vi "DAQ signal generation vi2.vi"(6 "Time for each step":dbl, 9 "Total time":dbl, 10 "DAQ1":waveform(dbl)[](array[waveform]), 11 "DAQ 2":waveform(dbl)[](array[waveform])) -> (0 "error out":errorcluster, 3 "error out 7":errorcluster)   [LabVIEW 2016]
uses:
  <vilib>/DAQmx/write.llb/DAQmx Write (Analog 1D Wfm NChan NSamp).vi
  <vilib>/DAQmx/create/channels.llb/DAQmx Create Channel (AO-Voltage-Basic).vi
  <vilib>/DAQmx/configure/timing.llb/DAQmx Timing (Sample Clock).vi
  <vilib>/DAQmx/miscellaneous.llb/DAQmx Fill In Error Info.vi
  <vilib>/DAQmx/configure/trigger.llb/DAQmx Start Trigger (Digital Edge).vi
  <resource>/objmgr/daqmx.rc
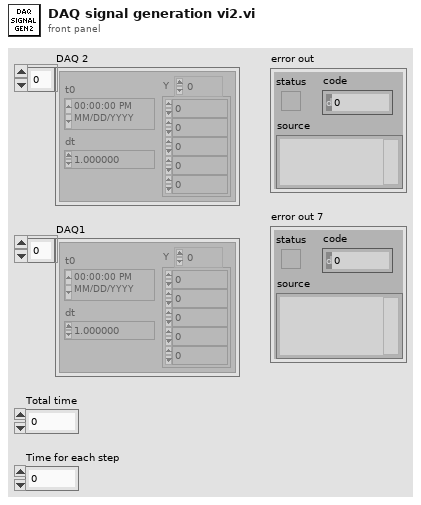
[diagram p1: front panel]
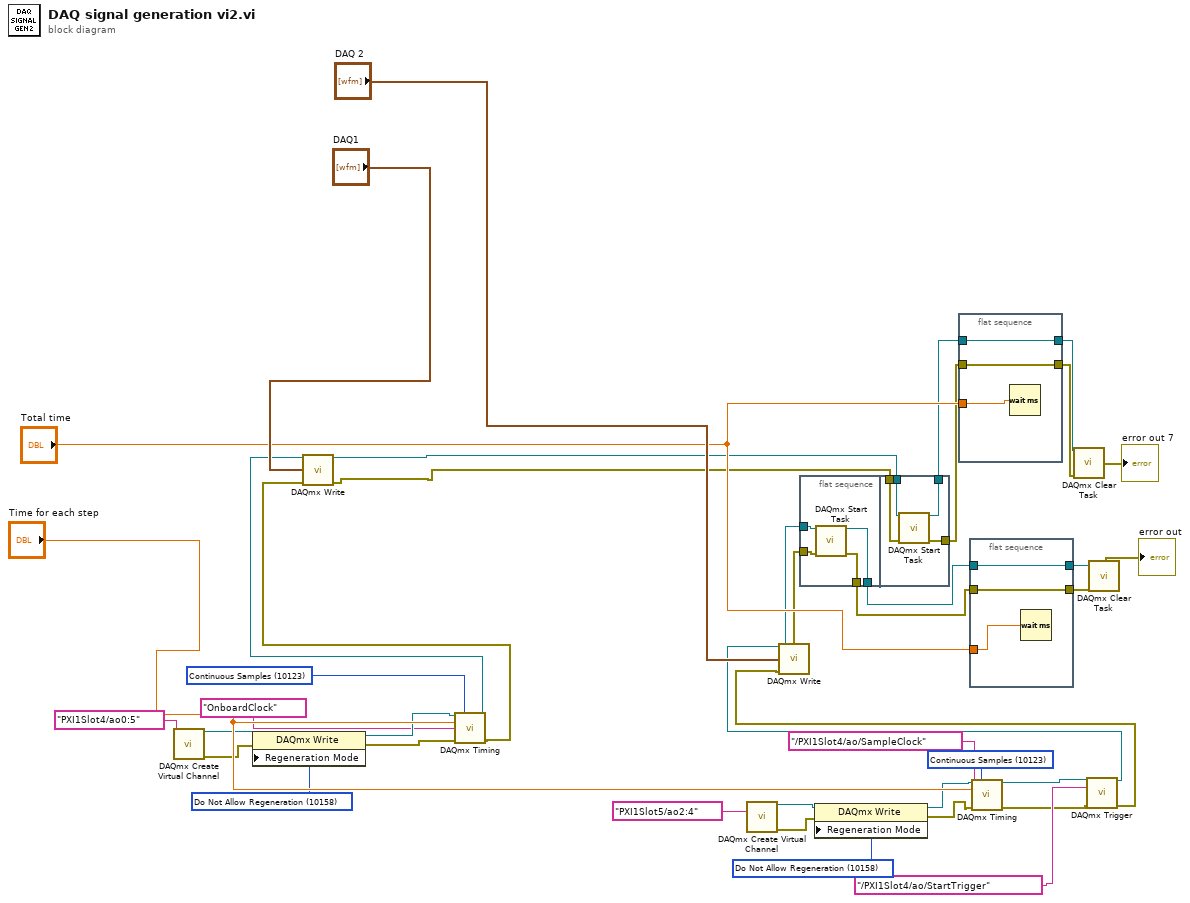
[diagram p0: block diagram]
diagram:
  w37 = 10158 items=["Allow Regeneration"=10097, "Do Not Allow Regeneration"=10158] ("RegenMode")
  w11 = 10158 items=["Allow Regeneration"=10097, "Do Not Allow Regeneration"=10158] ("RegenMode")
  w10 = 10123 items=["Finite Samples"=10178, "Continuous Samples"=10123, "Hardware Timed Single Point"=12522] ("sample mode")
  w4 = 10123 items=["Finite Samples"=10178, "Continuous Samples"=10123, "Hardware Timed Single Point"=12522] ("sample mode")
  n1 = call-poly <vilib>:"DAQmx Create Virtual Channel.vi"("physical channels"=tag "PXI1Slot4/ao0:5") -> ("task out"=w35:refnum<k21>, "error out"=w36:errorcluster)  [unwired: 13 in]
  n2 = property class="DAQmx Write"(reference=w35, error in=w36, "Regeneration Mode"=w37) -> (reference out=w33:refnum<k21>, error out=w34:errorcluster)
  n3 = call-poly <vilib>:"DAQmx Timing.vi"("task/channels in"=w33, "sample mode"=w4, "rate"="Time for each step", "source"=tag "OnboardClock", "error in"=w34) -> ("task out"=w5:refnum<k21>, "error out"=w32:errorcluster)  [unwired: 9 in]
  n4 = call-poly <vilib>:"DAQmx Write.vi"("task/channels in"=w5, "data"="DAQ1", "error in"=w32) -> ("task out"=w26:refnum<k21>, "error out"=w27:errorcluster)  [unwired: 10 in, 1 out]
  n5 = call-poly <vilib>:"DAQmx Create Virtual Channel.vi"("physical channels"=tag "PXI1Slot5/ao2:4") -> ("task out"=w6:refnum<k21>, "error out"=w7:errorcluster)  [unwired: 13 in]
  n6 = flat-sequence {
    tunnel: w17 -> [w45]
    tunnel: w18 -> [w44]
    tunnel: [w43] -> w23
    tunnel: [w42] -> w24
    tunnel: w26 -> [w49]
    tunnel: w27 -> [w48]
    tunnel: [w47] -> w28
    tunnel: [w46] -> w31
    frame #0 {
      n7 = call <vilib>:"DAQmx Start Task.vi"("task/channels in"=w44, "error in"=w45) -> ("task out"=w42:refnum<k21>, "error out"=w43:errorcluster)  [unwired: 12 in]
    }
    frame #1 {
      n8 = call <vilib>:"DAQmx Start Task.vi"("task/channels in"=w49, "error in"=w48) -> ("task out"=w47:refnum<k21>, "error out"=w46:errorcluster)  [unwired: 12 in]
    }
  }
  n9 = property class="DAQmx Write"(reference=w6, error in=w7, "Regeneration Mode"=w11) -> (reference out=w8:refnum<k21>, error out=w9:errorcluster)
  n10 = flat-sequence {
    tunnel: w31 -> [w51]
    tunnel: w28 -> [w52]
    tunnel: [w52] -> w29
    tunnel: [w51] -> w30
    tunnel: "Total time" -> [w50]
    frame #0 {
      n11 = Wait (ms)(milliseconds to wait=w50) -> ()  [unwired: 1 out]
    }
  }
  n12 = flat-sequence {
    tunnel: w23 -> [w54]
    tunnel: w24 -> [w55]
    tunnel: [w55] -> w19
    tunnel: [w54] -> w20
    tunnel: "Total time" -> [w53]
    frame #0 {
      n13 = Wait (ms)(milliseconds to wait=w53) -> ()  [unwired: 1 out]
    }
  }
  n14 = call-poly <vilib>:"DAQmx Timing.vi"("task/channels in"=w8, "sample mode"=w10, "rate"="Time for each step", "source"=tag "/PXI1Slot4/ao/SampleClock", "error in"=w9) -> ("task out"=w12:refnum<k21>, "error out"=w13:errorcluster)  [unwired: 9 in]
  n15 = call <vilib>:"DAQmx Clear Task.vi"("task in"=w29, "error in"=w30) -> ("error out"=→"error out 7":errorcluster)  [unwired: 13 in]
  n16 = call-poly <vilib>:"DAQmx Trigger.vi"("task/channels in"=w12, "source"=tag "/PXI1Slot4/ao/StartTrigger", "error in"=w13) -> ("task out"=w21:refnum<k21>, "error out"=w22:errorcluster)  [unwired: 11 in]
  n17 = call-poly <vilib>:"DAQmx Write.vi"("task/channels in"=w21, "data"="DAQ 2", "error in"=w22) -> ("task out"=w18:refnum<k21>, "error out"=w17:errorcluster)  [unwired: 10 in, 1 out]
  n18 = call <vilib>:"DAQmx Clear Task.vi"("task in"=w19, "error in"=w20) -> ("error out"=→"error out":errorcluster)  [unwired: 13 in]
